vi "Setup.vi"(11 "Sound Demo.lvclass":refnum<class "Sound Demo.lvclass">) -> (0 "error out":errorcluster, 3 "Sound Demo.lvclass out":refnum<class "Sound Demo.lvclass">)   [LabVIEW 2010, in "Sound Demo.lvclass"]
doc: "Select which sound player should be used for the demo."
uses:
  Sound Demo.lvclass
  Sound Visualizer/Sound Visualizer.lvclass
  Sound Demo.lvclass/Sound Demo.ctl
panel:
  in  "Cancel":bool
  in  "OK":bool
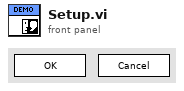
[diagram p1: front panel]
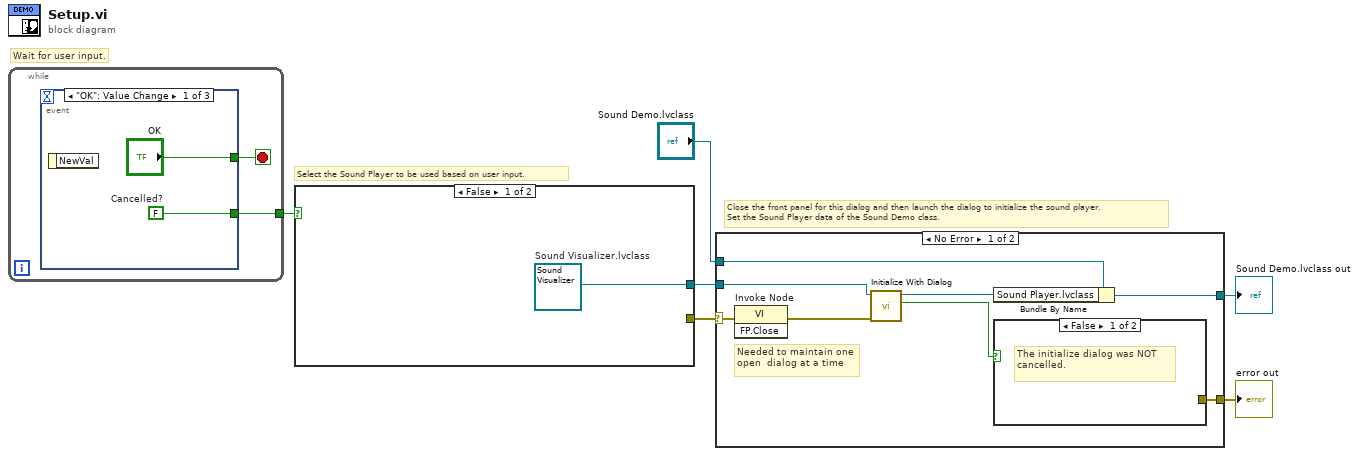
[diagram p0: block diagram]
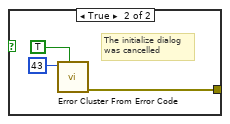
[diagram p2: hidden frame]
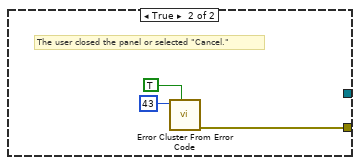
[diagram p4: hidden frame]
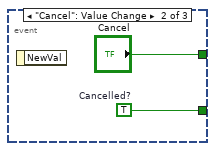
[diagram p5: hidden frame]
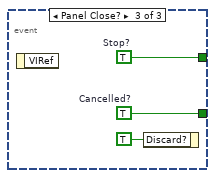
[diagram p6: hidden frame]
diagram:
  # "Close the front panel for this dialog and then launch the dialog to initialize the sound player.\nSet the Sound Player data of the Sound Demo class."
  # "Select the Sound Player to be used based on user input."
  # "Wait for user input."
  n1 = while {
    tunnel: [w7] -> w6
    stop <- w8 stop-if-true
    n2 = event shown="[0] \"OK\": Value Change" {
      selector: _ -> [_ _ _]
      dyn-events: _ -> [_ _ _]
      timeout: _ -> [_ _ _]
      tunnel: ["OK" "Cancel" w14] -> w8
      tunnel: [w10 w12 w13] -> w7
      event "OK": Value Change {
        w10 = FALSE  # Cancelled?
        n3 = event-data() -> ()  [unwired: 1 in, 1 out]
      }
      event "Cancel": Value Change {
        w12 = TRUE  # Cancelled?
        n4 = event-data() -> ()  [unwired: 1 in, 1 out]
      }
      event Panel Close? {
        w13 = TRUE  # Cancelled?
        w14 = TRUE  # Stop?
        n5 = event-data() -> ()  [unwired: 1 in, 1 out]
        n6 = event-data("Discard?"=TRUE) -> ()  [unwired: 1 in, 1 out]
      }
    }
  }
  n7 = case shown="False" w6 {
    tunnel: [_ w17] -> w5
    tunnel: [w16 _] -> w4
    frame False {
      w16 = refnum<class "Sound Visualizer.lvclass"> refnum  # Sound Visualizer.lvclass
    }
    frame True {
      # "The user closed the panel or selected \"Cancel.\""
      n8 = call <vilib>:"Error Cluster From Error Code.vi"("show call chain? (False)"=TRUE, "error code (0)"=43) -> ("error out"=w17:errorcluster)  [unwired: 7 in]
    }
  }
  n9 = case shown="No Error" w5 {
    selector: w5 -> [w21 w31]
    tunnel: w4 -> [w27 _]
    tunnel: "Sound Demo.lvclass" -> [w25 w32]
    tunnel: [w24 w32] -> w2
    tunnel: [w22 w31] -> w1
    frame No Error {
      # "Needed to maintain one open  dialog at a time"
      n10 = invoke on="Invoke Node" class="VI" method="FP.Close"(error in=w21) -> (error out=w20:errorcluster)  [unwired: 2 in, 2 out]
      n11 = call-dynamic "Initialize With Dialog.vi"("error in (no error)"=w20, "Sound Player in"=w27) -> ("Cancelled?"=w23:bool, "Sound Player out"=w26:refnum<class "Sound Visualizer.lvclass">)  [unwired: 7 in, 1 out]
      n12 = Bundle By Name "Bundle By Name"(cluster=w25, "Sound Player.lvclass"=w26) -> (w24:refnum<class "Sound Demo.lvclass">)
      n13 = case shown="False" w23 {
        tunnel: [_ w28] -> w22
        frame False {
          # "The initialize dialog was NOT cancelled."
        }
        frame True {
          # "The initialize dialog\nwas cancelled"
          n14 = call <vilib>:"Error Cluster From Error Code.vi"("show call chain? (False)"=TRUE, "error code (0)"=43) -> ("error out"=w28:errorcluster)  [unwired: 7 in]
        }
      }
    }
    frame Error {
    }
  }
  "Sound Demo.lvclass out" <- w2
  "error out" <- w1
